vi "Process.vi"(8 "error in":errorcluster, 11 "SMO":refnum<class "SMO.lvclass">) -> (0 "error out":errorcluster, 3 "SMO out":refnum<class "SMO.lvclass">)   [LabVIEW 2019, in "SMO.lvclass"]
doc: "JKI State Machine Objects (SMO) 1.3.0.56\nJKI - JKI\nCopyright (c) 2017, JKI"
uses:
  SMO.lvclass
  Typedefs/SMOState --Enum.ctl
  Support/Attribute.Owner/Packet -- Cluster.ctl
  Typedefs/Parent Call--Enum.ctl
  SMO.lvclass/SMO.ctl
  Typedefs/Search Key.ctl
  Support/Attribute.Owner/Attribute.Owner.lvclass
panel:
  in  "Test Error":bool
  # "For instructions on how to use the JKI State Machine Objects, examples and video tutorials, visit:\nhttp://jki.net/state-machine-objects/\n\nJKI State Machine Objects™\nhttp://jki.net/state-machine-objects/\nCopyright (C) 2005-2015, JKI <info@jki.net>\nALL RIGHTS RESERVED"
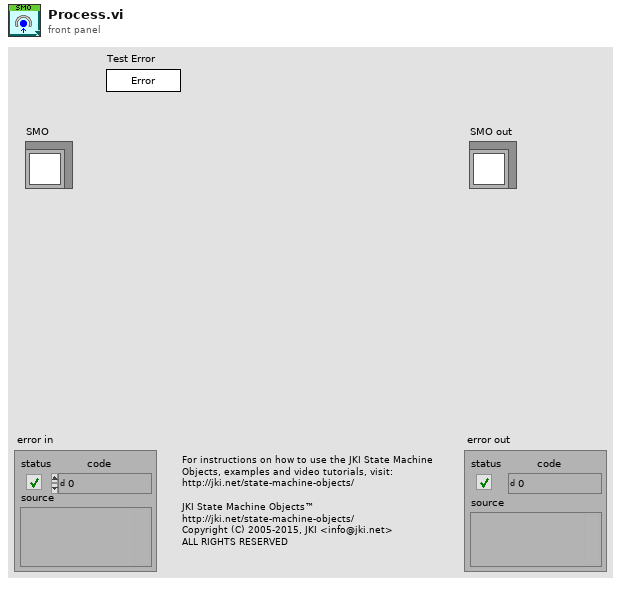
[diagram p1: front panel]
types:
  T1 = typedef "SMO.lvclass/Parent Call--Enum.ctl" = enum16{"Allows parent to run", "Does not request parent to run"}
  T2 = typedef "SMO.lvclass/Protected Events.ctl" = cluster{"StopProcesses":refnum<user-event>, "AbortProcesses":refnum<user-event>, "Config Changed":refnum<user-event>, "Dependency":refnum<user-event>}
  T3 = typedef "SMO.lvclass/Public Events.ctl" = cluster{"Error":refnum<user-event>, "State":refnum<user-event>, "Reserve State":refnum<user-event>}
  T4 = typedef "SMO.lvclass/SMOState --Enum.ctl" = enum16{"unknown", "Created", "Started", "Stopped"}
  T5 = typedef "Attribute.Owner.lvclass/Packet -- Cluster.ctl" = cluster{"Message":string, "Payload":variant, "Source GUID":string}
  T6 = typedef "SMO.lvclass/Search Key.ctl" = enum16{"Name", "GUID", "Qualified Name", "Subsystem Path", "Configuration Path"}
  T7 = cluster{"[Dependencies]":refnum<class "SMO.lvclass">[], "State [Dependencies]":refnum<user-event>[], "Error [Dependencies]":refnum<user-event>[], "Message [Dependencies]":refnum<user-event>[]}
  T8 = typedef "SMO.lvclass/SMO Dependency Event--Enum.ctl" = enum16{"Added", "Removed", "Started", "Stopped"}
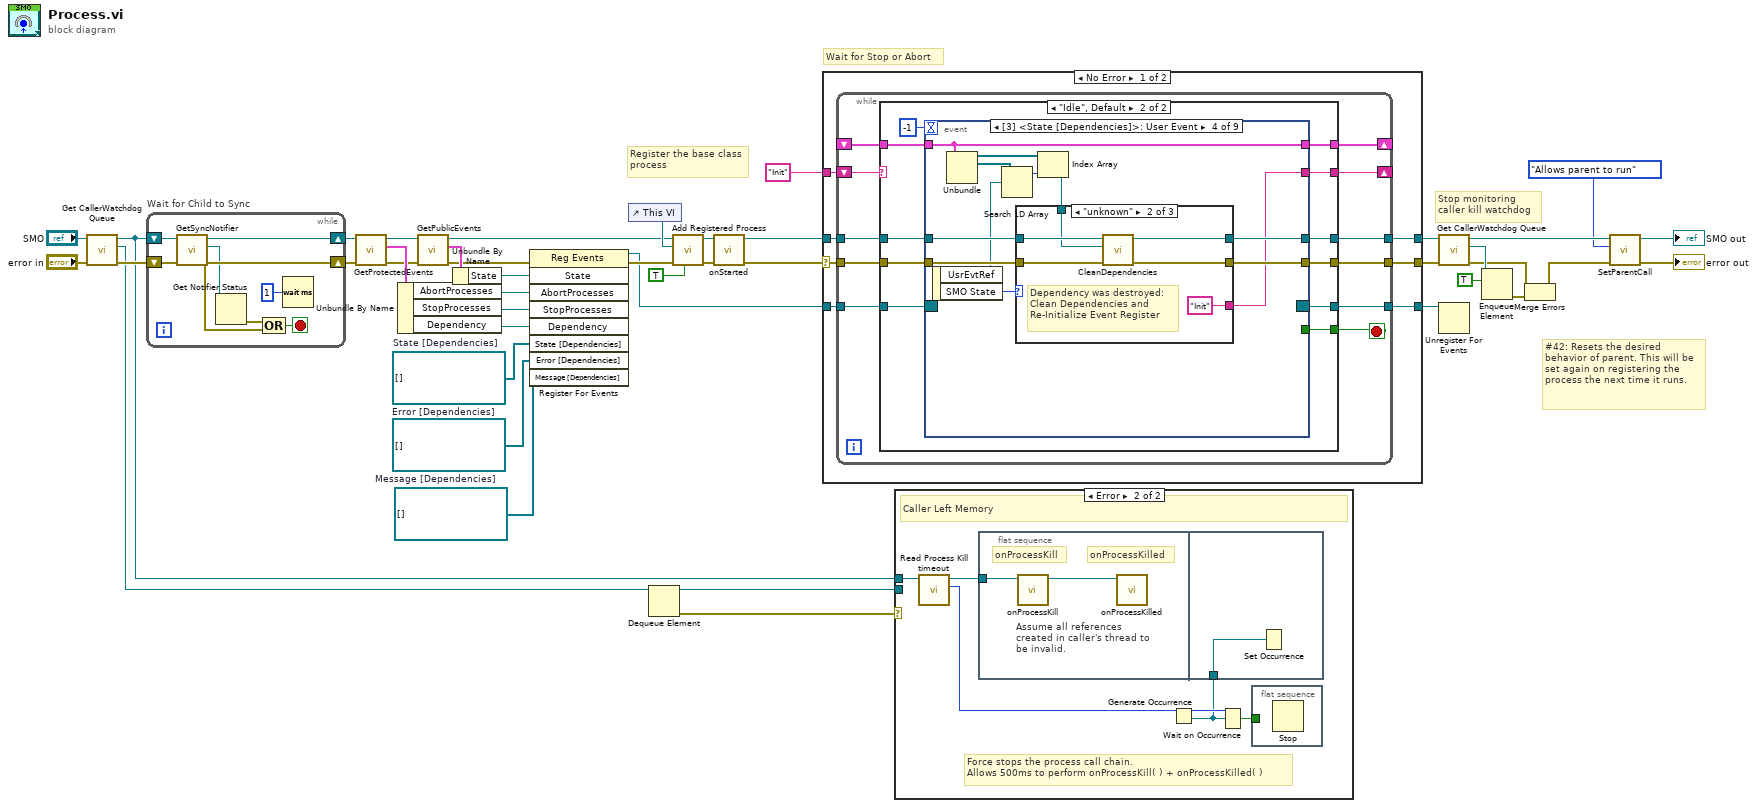
[diagram p0: block diagram]
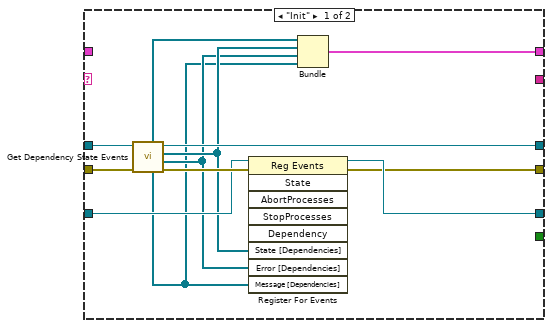
[diagram p3: hidden frame]
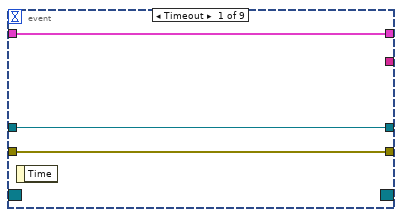
[diagram p4: hidden frame]
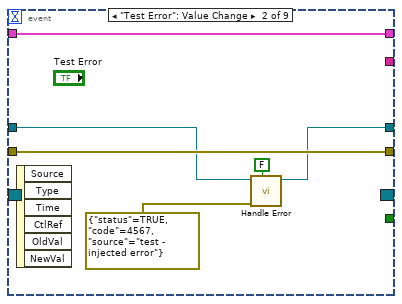
[diagram p5: hidden frame]
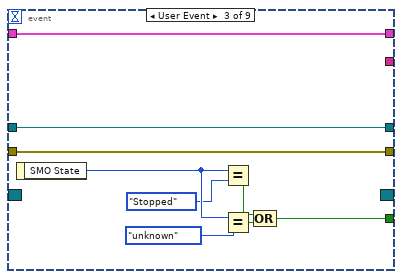
[diagram p6: hidden frame]
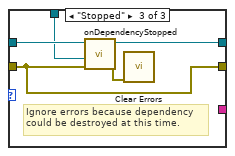
[diagram p8: hidden frame]
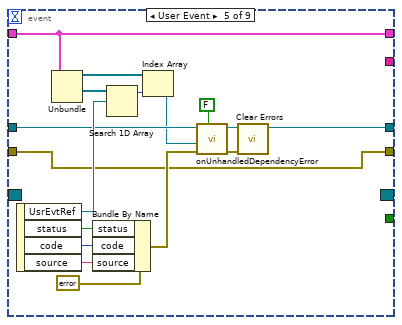
[diagram p9: hidden frame]
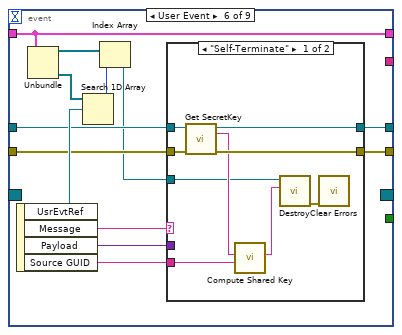
[diagram p10: hidden frame]
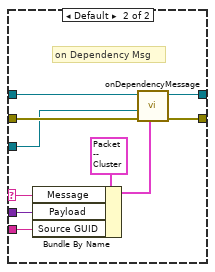
[diagram p11: hidden frame]
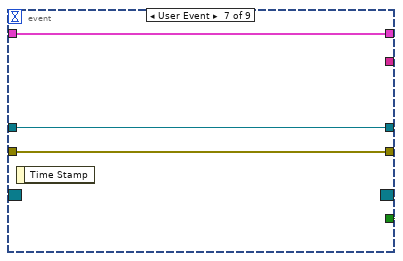
[diagram p12: hidden frame]
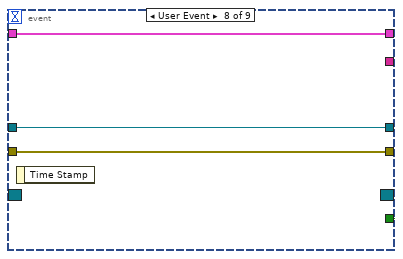
[diagram p13: hidden frame]
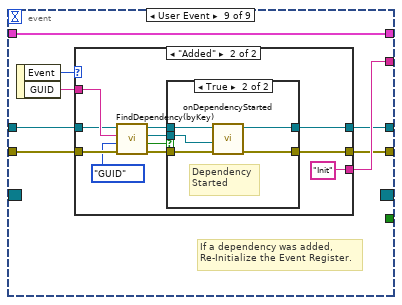
[diagram p14: hidden frame]
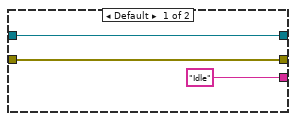
[diagram p15: hidden frame]
diagram:
  w6 = refnum<user-event>[] []  # Message [Dependencies]
  w11 = refnum<user-event>[] []  # Error [Dependencies]
  w14 = refnum<user-event>[] [] items=["unknown", "Created", "Started", "Stopped"]  # State [Dependencies]
  # "#42: Resets the desired behavior of parent. This will be set again on registering the process the next time it runs."
  # "Stop monitoring\ncaller kill watchdog"
  # "Wait for Stop or Abort"
  # "Register the base class\nprocess"
  n1 = call "Get CallerWatchdog Queue.vi"("error in (no error)"="error in", "SMO in"="SMO") -> ("error out"=w18:errorcluster, "Caller Watchdog"=w17:refnum<queue>, "SMO out"=w16:refnum<class "SMO.lvclass">)  [unwired: 7 in]
  n2 = while "Wait for Child to Sync" {
    shift-right: [w50] -> w13
    shift-left: w16 -> [w51]
    shift-right: [w47] -> w12
    shift-left: w18 -> [w49]
    stop <- w48 stop-if-true
    n3 = call "GetSyncNotifier.vi"("error in (no error)"=w49, "SMO in"=w51) -> ("error out"=w47:errorcluster, "Sync Notifier"=w45:refnum<notifier>, "SMO out"=w50:refnum<class "SMO.lvclass">)  [unwired: 7 in]
    n4 = Get Notifier Status(notifier=w45) -> (error out=w44:errorcluster)  [unwired: 1 in, 4 out]
    n5 = Compound Arithmetic op=OR(w44, w47) -> (w48:bool)
    n6 = Wait (ms)(milliseconds to wait=u32 1) -> ()  [unwired: 1 out]
  }
  n7 = call "GetProtectedEvents.vi"("error in (no error)"=w12, "SMO"=w13) -> ("error out"=w38:errorcluster, "SMO Protected Events"=w41:T2, "SMO out"=w39:refnum<class "SMO.lvclass">)  [unwired: 7 in]
  n8 = Unbundle By Name(w41) -> ("AbortProcesses"=w42:refnum<user-event>, "StopProcesses"=w36:refnum<user-event>, "Dependency"=w15:refnum<user-event>)
  n9 = call "GetPublicEvents.vi"("error in (no error)"=w38, "SMO"=w39) -> ("error out"=w37:errorcluster, "Public Events"=w40:T3, "SMO out"=w30:refnum<class "SMO.lvclass">)  [unwired: 7 in]
  n10 = Unbundle By Name(w40) -> ("State"=w43:refnum<user-event>)
  n11 = register-events(error in=w37, w43, w42, w36, w15, w14, w11, w6) -> (reference out=w9:refnum<event-registration>, error out=w29:errorcluster)  [unwired: 1 in]
  n12 = control-ref of="This VI"() -> (w34:refnum<vi>)
  n13 = Dequeue Element(queue=w17) -> (queue out=w23:refnum<queue>, error out=w24:errorcluster)  [unwired: 2 in, 2 out]
  n14 = call "Add Registered Process.vi"("Process Runs (T)"=TRUE, "error in (no error)"=w29, "Process VI (Static VI Ref)"=w34, "SMO"=w30) -> ("error out"=w31:errorcluster, "SMO out"=w32:refnum<class "SMO.lvclass">)  [unwired: 6 in]
  n15 = call-dynamic "onStarted.vi"("error in (no error)"=w31, "SMO"=w32) -> ("error out"=w8:errorcluster, "SMO out"=w7:refnum<class "SMO.lvclass">)  [unwired: 8 in]
  n16 = case shown="No Error" w8 {
    selector: w8 -> [w56 w223]
    tunnel: [w58 w223] -> w28
    tunnel: w9 -> [w57 w222]
    tunnel: [w55 w222] -> w35
    tunnel: w7 -> [w54 w221]
    tunnel: [w53 w221] -> w27
    tunnel: "Init" -> [w52 _]
    frame No Error {
      n17 = while {
        tunnel: [w69] -> w58
        tunnel: w57 -> [w68]
        tunnel: w56 -> [w67]
        tunnel: [w66] -> w55
        tunnel: w54 -> [w65]
        tunnel: [w64] -> w53
        shift-right: [w62] -> _
        shift-left: w52 -> [w61]
        shift-right: [w60] -> _
        shift-left: _ -> [w59]
        stop <- w63 stop-if-true
        n18 = case shown="\"Idle\", Default" w61 {
          tunnel: [w76 w92] -> w69
          tunnel: w68 -> [w78 w91]
          tunnel: w67 -> [w75 w90]
          tunnel: [w77 w89] -> w66
          tunnel: w65 -> [w80 w88]
          tunnel: [w79 w87] -> w64
          tunnel: [_ w85] -> w63
          tunnel: [_ w84] -> w62
          tunnel: [w71 w82] -> w60
          tunnel: w59 -> [_ w83]
          frame "Init" {
            n19 = call "Get Dependency State Events.vi"("error in (no error)"=w75, "SMO in"=w80) -> ("error out"=w81:errorcluster, "Error [Dependencies]"=w72:refnum<user-event>[], "State [Dependencies]"=w73:refnum<user-event>[], "SMO out"=w79:refnum<class "SMO.lvclass">, "Message [Dependencies]"=w70:refnum<user-event>[], "[Dependencies]"=w74:refnum<class "SMO.lvclass">[])  [unwired: 4 in]
            n20 = register-events(reference=w78, error in=w81, w73, w72, w70) -> (reference out=w77:refnum<event-registration>, error out=w76:errorcluster)  [unwired: 4 in]
            n21 = Bundle("[Dependencies]"=w74, "State [Dependencies]"=w73, "Error [Dependencies]"=w72, "Message [Dependencies]"=w70) -> (w71:T7)  [unwired: 1 in]
          }
          frame "Idle", Default {
            n22 = event shown="[3] <State [Dependencies]>: User Event" {
              selector: w91 -> [_ _ _ _ _ _ _ _ _]
              dyn-events: [_ _ _ _ _ _ _ _ _] -> w89
              timeout: -1 -> [_ _ _ _ _ _ _ _ _]
              tunnel: w90 -> [w94 w101 w110 w118 w138 w156 w186 w190 w193]
              tunnel: [w94 w101 w110 w119 w138 w155 w186 w190 w194] -> w92
              tunnel: w88 -> [w95 w97 w106 w121 w142 w158 w187 w191 w196]
              tunnel: [w95 w96 w106 w120 w141 w157 w187 w191 w195] -> w87
              tunnel: [_ _ w103 _ _ _ TRUE TRUE _] -> w85
              tunnel: [_ _ _ w117 _ _ _ _ w197] -> w84
              tunnel: w83 -> [w93 w100 w102 w114 w147 w164 w184 w188 w199]
              tunnel: [w93 w100 w102 w114 w147 w164 w184 w188 w199] -> w82
              event Timeout {
                n23 = event-data() -> ()  [unwired: 1 in, 1 out]
              }
              event "Test Error": Value Change {
                n24 = event-data() -> ()  [unwired: 1 in, 6 out]
                n25 = call-dynamic "Handle Error.vi"("Stop on Unhandled Error (T)"=FALSE, "error in"=errorcluster {"status"=TRUE, "code"=4567, "source"="test - injected error"}, "SMO"=w97) -> ("SMO out"=w96:refnum<class "SMO.lvclass">)  [unwired: 6 in, 2 out]
              }
              event User Event {
                n26 = event-data() -> ("SMO State"=w105:T4)  [unwired: 1 in]
                n27 = Equal?(x=w105, y=SMOState_--Enum."Stopped") -> (x = y?=w108:bool)
                n28 = Equal?(x=w105, y=SMOState_--Enum."unknown") -> (x = y?=w109:bool)
                n29 = Compound Arithmetic op=OR(w108, w109) -> (w103:bool)
              }
              event User Event {
                n30 = event-data() -> ("UsrEvtRef"=w112:refnum<user-event>, "SMO State"=w122:T4)  [unwired: 1 in]
                n31 = Unbundle(w114) -> ("[Dependencies]"=w115:refnum<class "SMO.lvclass">[], "State [Dependencies]"=w113:refnum<user-event>[])  [unwired: 2 out]
                n32 = Search 1D Array(1D array=w113, element=w112) -> (index of element=w116:i32)  [unwired: 1 in]
                n33 = Index Array(array=w115, index=w116) -> (element=w111:refnum<class "SMO.lvclass">)
                n34 = case shown="\"unknown\"" w122 {
                  tunnel: w121 -> [w124 w130 w135]
                  tunnel: [w124 w129 w133] -> w120
                  tunnel: [w123 w127 w132] -> w119
                  tunnel: w118 -> [w123 w128 w132]
                  tunnel: [_ "Init" _] -> w117
                  tunnel: w111 -> [_ w125 w134]
                  frame Default {
                  }
                  frame "unknown" {
                    # "Dependency was destroyed:\nClean Dependencies and\nRe-Initialize Event Register"
                    n35 = call "CleanDependencies.vi"("error in (no error)"=w128, "Dependency"=w125, "SMO in"=w130) -> ("error out"=w127:errorcluster, "SMO out"=w129:refnum<class "SMO.lvclass">)  [unwired: 6 in, 1 out]
                  }
                  frame "Stopped" {
                    # "Ignore errors because dependency\ncould be destroyed at this time."
                    n36 = call-dynamic "onDependencyStopped.vi"("error in"=w132, "Dependency"=w134, "SMO in"=w135) -> ("error out"=w131:errorcluster, "SMO out"=w133:refnum<class "SMO.lvclass">)  [unwired: 7 in]
                    n37 = call <vilib>:"Clear Errors.vi"("error in (no error)"=w131) -> ()  [unwired: 5 in, 2 out]
                  }
                }
              }
              event User Event {
                n38 = event-data() -> ("UsrEvtRef"=w145:refnum<user-event>, "status"=w148:bool, "code"=w149:i32, "source"=w150:string)  [unwired: 1 in]
                n39 = Unbundle(w147) -> ("[Dependencies]"=w144:refnum<class "SMO.lvclass">[], "Error [Dependencies]"=w146:refnum<user-event>[])  [unwired: 2 out]
                n40 = Bundle By Name(cluster=errorcluster {"status"=FALSE, "code"=0, "source"=""} ("error constant"), "status"=w148, "code"=w149, "source"=w150) -> (w140:errorcluster)
                n41 = Search 1D Array(1D array=w146, element=w145) -> (index of element=w143:i32)  [unwired: 1 in]
                n42 = Index Array(array=w144, index=w143) -> (element=w139:refnum<class "SMO.lvclass">)
                n43 = call-dynamic "onUnhandledDependencyError.vi"("Stop on Unhandled Error (F)"=FALSE, "Unhandled Dependency Error"=w140, "Dependency"=w139, "SMO in"=w142) -> ("Unhandled error"=w136:errorcluster, "SMO out"=w141:refnum<class "SMO.lvclass">)  [unwired: 6 in]
                n44 = call <vilib>:"Clear Errors.vi"("error in (no error)"=w136) -> ()  [unwired: 5 in, 2 out]
              }
              event User Event {
                n45 = event-data() -> ("UsrEvtRef"=w163:refnum<user-event>, "Message"=w159:string, "Payload"=w152:variant, "Source GUID"=w153:string)  [unwired: 1 in]
                n46 = Unbundle(w164) -> ("[Dependencies]"=w162:refnum<class "SMO.lvclass">[], "Message [Dependencies]"=w160:refnum<user-event>[])  [unwired: 2 out]
                n47 = Search 1D Array(1D array=w160, element=w163) -> (index of element=w161:i32)  [unwired: 1 in]
                n48 = Index Array(array=w162, index=w161) -> (element=w154:refnum<class "SMO.lvclass">)
                n49 = case shown="\"Self-Terminate\"" w159 {
                  selector: w159 -> [_ w176]
                  tunnel: w158 -> [w173 w183]
                  tunnel: [w172 w182] -> w157
                  tunnel: w156 -> [w171 w181]
                  tunnel: [w170 w180] -> w155
                  tunnel: w154 -> [w167 w179]
                  tunnel: w153 -> [w169 w174]
                  tunnel: w152 -> [_ w175]
                  frame "Self-Terminate" {
                    n50 = call "Get SecretKey.vi"("error in (no error)"=w171, "SMO"=w173) -> ("error out"=w170:errorcluster, "SecretKey"=w168:string, "SMO out"=w172:refnum<class "SMO.lvclass">)  [unwired: 7 in]
                    n51 = call "Compute Shared Key.vi"("GUID"=w169, "SecretKey"=w168) -> ("Shared Key"=w166:string)  [unwired: 9 in]
                    n52 = call "Destroy.vi"("Shared Key"=w166, "SMO"=w167) -> ("error out"=w165:errorcluster)  [unwired: 9 in]
                    n53 = call <vilib>:"Clear Errors.vi"("error in (no error)"=w165) -> ()  [unwired: 5 in, 2 out]
                  }
                  frame Default {
                    # "on Dependency Msg"
                    n54 = Bundle By Name(cluster=T5 {"Message"="", "Payload"=variant, "Source GUID"=""} ("Packet"), "Message"=w176, "Payload"=w175, "Source GUID"=w174) -> (w178:T5)
                    n55 = call-dynamic "onDependencyMessage.vi"("Packet"=w178, "error in"=w181, "Dependency"=w179, "SMO in"=w183) -> ("error out"=w180:errorcluster, "SMO out"=w182:refnum<class "SMO.lvclass">)  [unwired: 6 in]
                  }
                }
              }
              event User Event {
                n56 = event-data() -> ()  [unwired: 1 in, 1 out]
              }
              event User Event {
                n57 = event-data() -> ()  [unwired: 1 in, 1 out]
              }
              event User Event {
                # "If a dependency was added,\nRe-Initialize the Event Register."
                n58 = event-data() -> ("Event"=w198:T8, "GUID"=w192:string)  [unwired: 1 in]
                n59 = case shown="\"Added\"" w198 {
                  tunnel: ["Idle" "Init"] -> w197
                  tunnel: w196 -> [w201 w211]
                  tunnel: [w201 w205] -> w195
                  tunnel: [w200 w204] -> w194
                  tunnel: w193 -> [w200 w210]
                  tunnel: w192 -> [_ w212]
                  frame Default {
                  }
                  frame "Added" {
                    n60 = call "FindDependency(byKey).vi"("error in (no error)"=w210, "Search Key (Name)"=Search_Key."GUID", "Key"=w212, "SMO in"=w211) -> ("error out"=w207:errorcluster, "Found?"=w208:bool, "Dependency"=w203:refnum<class "SMO.lvclass">, "SMO dup"=w206:refnum<class "SMO.lvclass">)  [unwired: 4 in]
                    n61 = case shown="True" w208 {
                      tunnel: w207 -> [w214 w217]
                      tunnel: w206 -> [w215 w220]
                      tunnel: [w215 w218] -> w205
                      tunnel: [w214 w216] -> w204
                      tunnel: w203 -> [_ w219]
                      frame False {
                      }
                      frame True {
                        # "Dependency\nStarted"
                        n62 = call-dynamic "onDependencyStarted.vi"("error in"=w217, "Dependency"=w219, "SMO in"=w220) -> ("error out"=w216:errorcluster, "SMO out"=w218:refnum<class "SMO.lvclass">)  [unwired: 7 in]
                      }
                    }
                  }
                }
              }
            }
          }
        }
      }
    }
    frame Error {
    }
  }
  n63 = case shown="Error" w24 {
    tunnel: w23 -> [_ _]
    tunnel: w16 -> [_ w227]
    frame No Error {
      # "Process Terminated Normally"
    }
    frame Error {
      # "Force stops the process call chain.\nAllows 500ms to perform onProcessKill( ) + onProcessKilled( )"
      # "Caller Left Memory"
      n64 = call "Read Process Kill timeout.vi"("SMO in"=w227) -> ("Process Kill timeout (ms)"=w225:i32, "SMO out"=w226:refnum<class "SMO.lvclass">)  [unwired: 9 in]
      n65 = flat-sequence {
        tunnel: w226 -> [w230]
        tunnel: w224 -> [w231]
        frame #0 {
          # "Assume all references created in caller's thread to be invalid."
          # "onProcessKilled"
          # "onProcessKill"
          n66 = call-dynamic "onProcessKill.vi"("SMO in"=w230) -> ("SMO out"=w229:refnum<class "SMO.lvclass">)  [unwired: 10 in]
          n67 = call-dynamic "onProcessKilled.vi"("SMO in"=w229) -> ()  [unwired: 11 in]
        }
        frame #1 {
          n68 = Set Occurrence(w231) -> ()
        }
      }
      n69 = Generate Occurrence() -> (w224:refnum<k4>)
      n70 = Wait on Occurrence(2:w224, 3:w225) -> (0:w228:bool)  [unwired: 1 in]
      n71 = flat-sequence {
        tunnel: w228 -> [_]
        frame #0 {
          n72 = Stop() -> ()  [unwired: 1 in]
        }
      }
    }
  }
  n73 = call "Get CallerWatchdog Queue.vi"("error in (no error)"=w28, "SMO in"=w27) -> ("error out"=w21:errorcluster, "Caller Watchdog"=w26:refnum<queue>, "SMO out"=w3:refnum<class "SMO.lvclass">)  [unwired: 7 in]
  n74 = Unregister For Events(event registration refnum=w35) -> ()  [unwired: 1 in, 1 out]
  n75 = Enqueue Element(queue=w26, element=TRUE) -> (error out=w22:errorcluster)  [unwired: 2 in, 2 out]
  n76 = Merge Errors(w21, w22) -> (w5:errorcluster)
  n77 = call "SetParentCall.vi"("error in (no error)"=w5, "Parent Call"=Parent_Call--Enum."Allows parent to run", "SMO in"=w3) -> ("error out"=→"error out":errorcluster, "SMO out"=→"SMO out":refnum<class "SMO.lvclass">)  [unwired: 7 in]
